vi "print LCD.vi"(7 "Numero de colunas":i32, 8 "Error In":errorcluster, 9 "Texto":string="Teste", 10 "Coluna/linha":u8[](array[numeric]), 11 "LINX Resource":T1) -> (0 "Error Out":errorcluster, 3 "LINX Resource 2":T1)   [LabVIEW 2021]
uses:
  <vilib>/MakerHub/LINX/Private/Type Defs/LINX Ref.ctl
  <vilib>/MakerHub/LINX/Private/Type Defs/Platform.ctl
  <vilib>/MakerHub/LINX/Private/Type Defs/Interface.ctl
  <vilib>/MakerHub/LINX/Private/Device/Type Defs/LINX Device Config.ctl
  <vilib>/MakerHub/LINX/Private/Device/Type Defs/TCP Config.ctl
  <vilib>/MakerHub/LINX/Private/Device/Type Defs/Channels.ctl
  <vilib>/MakerHub/LINX/LMH-LINX.lvlib
  <vilib>/MakerHub/LINX/Private/Device/Device.lvlib
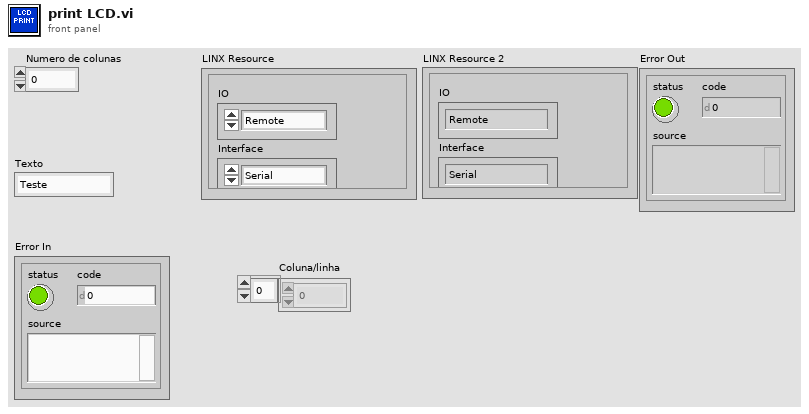
[diagram p1: front panel]
types:
  T1 = typedef "LMH-LINX.lvlib/LINX Ref.ctl" = cluster{"IO":T2, "Interface":T3, "LINX Device Config":T4}
  T2 = typedef "LMH-LINX.lvlib/Platform.ctl" = enum16{"Remote", "Local"}
  T3 = typedef "LMH-LINX.lvlib/Interface.ctl" = enum16{"Serial", "TCP"}
  T4 = typedef "LMH-LINX.lvlib/Device.lvlib/LINX Device Config.ctl" = cluster{"Interface":T3, "COM Port":refnum<visa-resource-name>, "TCP Configuration":T5, "Device Family":u8, "Device ID":u8, "Device Name":string, "TCP Ref":refnum<k5>, "Channels":T6}
  T5 = typedef "LMH-LINX.lvlib/Device.lvlib/TCP Config.ctl" = cluster{"IP Address":string, "Port":u16}
  T6 = typedef "LMH-LINX.lvlib/Channels.ctl" = cluster{"DI":u8[], "DO":u8[], "AI":u8[], "AO":u8[], "PWM":u8[], "QE":u8[], "UART":u8[], "I2C 2":u8[], "SPI":u8[], "CAN":u8[], "Servo":u8[], "AI Ref (V)":dbl, "AI Resolution (Bits)":u8, "AO Ref (V)":dbl, "AO Resolution (Bits)":u8}
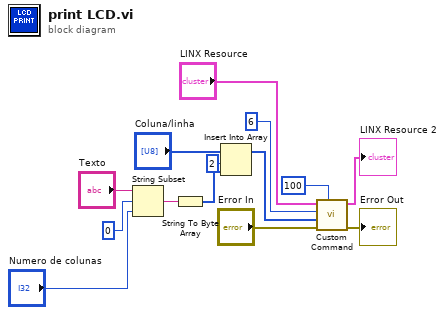
[diagram p0: block diagram]
diagram:
  n1 = String Subset(string="Texto", offset (0)=0, length (rest)="Numero de colunas") -> (substring=w11:string)
  n2 = String To Byte Array(string=w11) -> (unsigned byte array=w2:u8[])
  n3 = Insert Into Array(array="Coluna/linha", index=2, new element=w2) -> (w3:u8[])
  n4 = call <vilib>:"Custom Command.vi"("Timeout (100 ms)"=100, "Error In"="Error In", "Data"=w3, "Custom Command Number"=u16 6, "LINX Resource"="LINX Resource") -> ("Error Out"=→"Error Out":errorcluster, "LINX Resource"=→"LINX Resource 2":T1)  [unwired: 3 in, 2 out]
